vi "Parse Property Value.vi"(8 "error in":errorcluster, 10 "Property Type":T1, 11 "Node in":refnum<k20>) -> (0 "error out":errorcluster, 2 "Property Value":variant, 3 "Node out":refnum<k20>)   [LabVIEW 2024, in "Parser.lvlib" / "Property.lvclass"]
uses:
  Property.lvclass
  Controls/Property Type.ctl
  Controls/DependentFile.ctl
  <vilib>/xml/Close Reference(Node).vi
  <resource>/objmgr/DOMUserDefRef.rc
  <vilib>/xml/NI_XML.lvlib
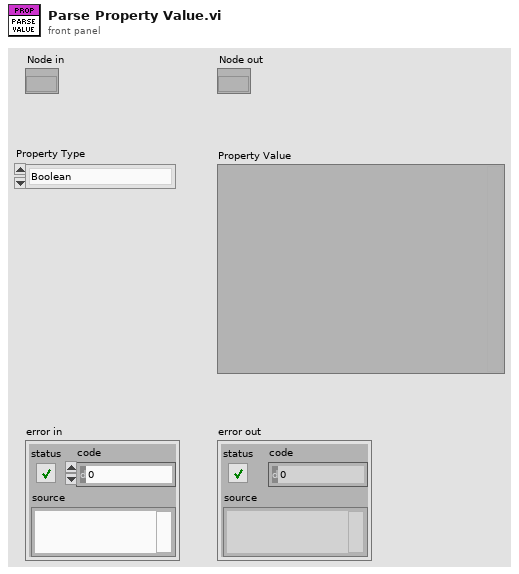
[diagram p1: front panel]
types:
  T1 = typedef "Parser.lvlib/Property.lvclass/Property Type.ctl" = enum16{"Boolean", "Double", "String", "Path", "Dictionary", "DependentFile", "I16", "I32", "I64", "U16", "U32", "U64", "BooleanArray", "DoubleArray", "StringArray", "I16Array", "I32Array", "I64Array", "U16Array", "U32Array", "U64Array", "Variant"}
  T2 = typedef "Parser.lvlib/Property.lvclass/DependentFile.ctl" = cluster{"Path":path, "Version":string, "RTDestination":path, "ForceDownload":bool, "SupportedTarget":string, "MD5":string, " Type":string}
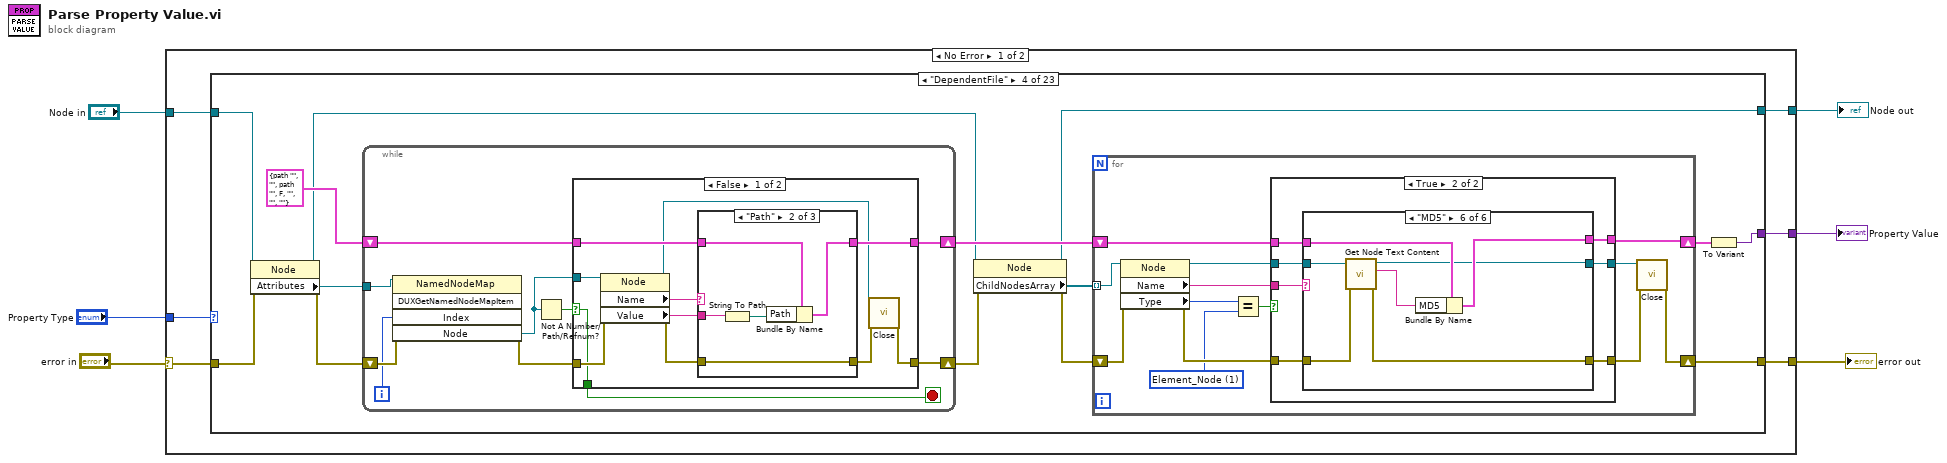
[diagram p0: block diagram]
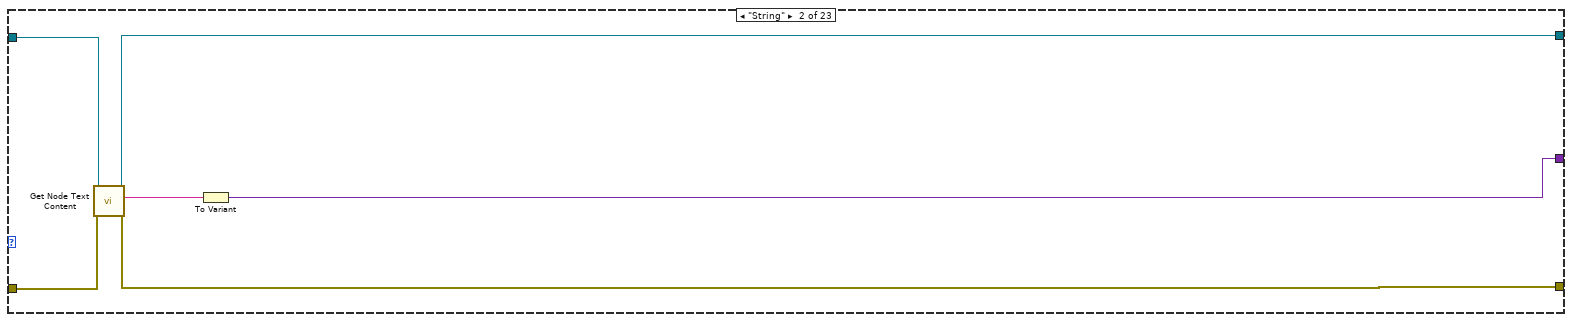
[diagram p3: hidden frame]
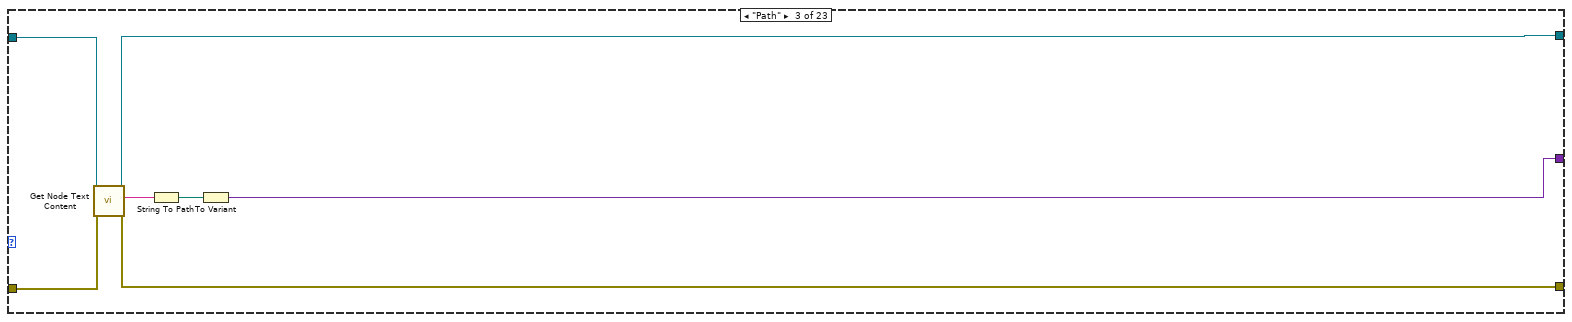
[diagram p4: hidden frame]
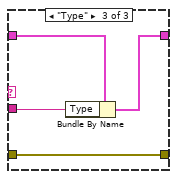
[diagram p6: hidden frame]
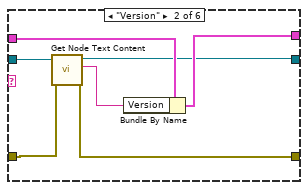
[diagram p10: hidden frame]
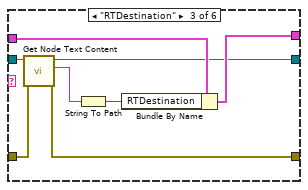
[diagram p11: hidden frame]
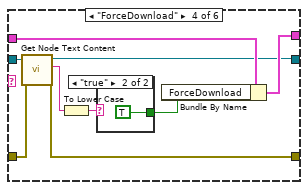
[diagram p12: hidden frame]
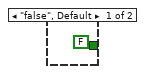
[diagram p13: hidden frame]
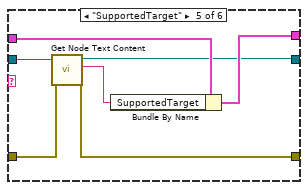
[diagram p14: hidden frame]
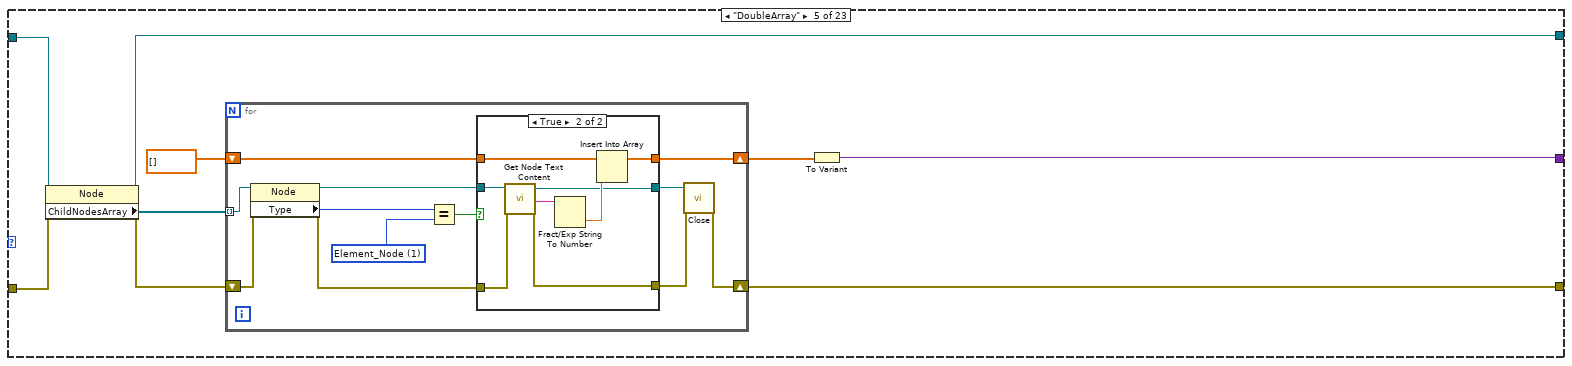
[diagram p15: hidden frame]
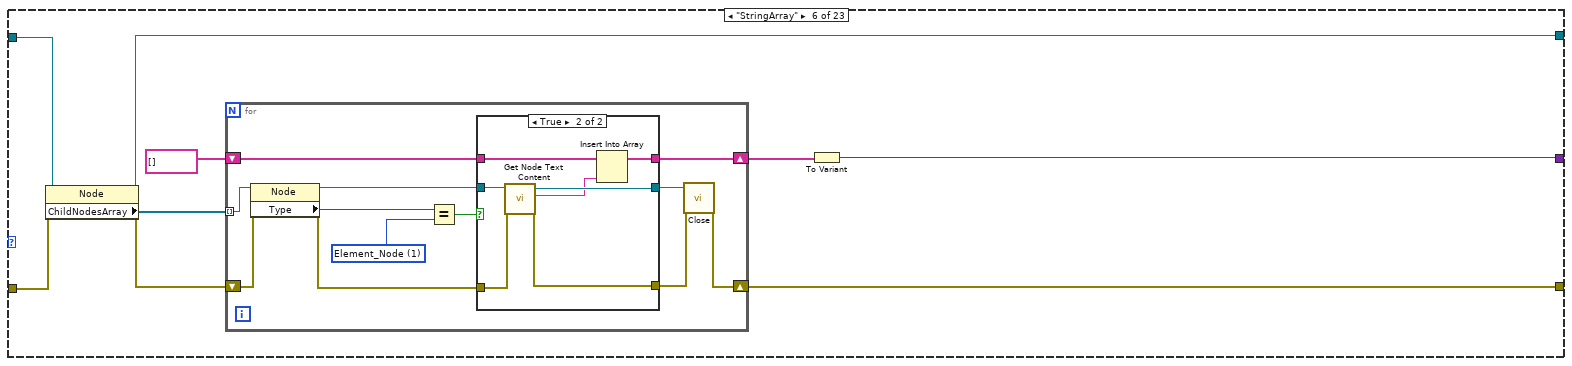
[diagram p17: hidden frame]
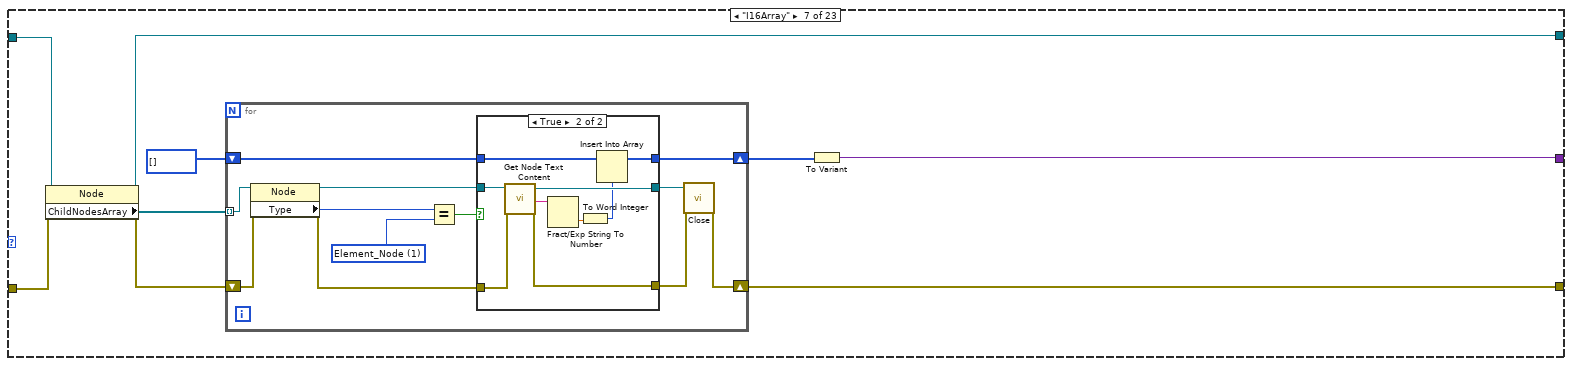
[diagram p19: hidden frame]
diagram:
  n1 = case shown="No Error" "error in" {
    selector: "error in" -> [w11 w608]
    tunnel: [w12 w608] -> w6
    tunnel: "Node in" -> [w10 w607]
    tunnel: [w9 _] -> w3
    tunnel: [w8 w607] -> w2
    tunnel: "Property Type" -> [w7 _]
    frame No Error {
      n2 = case shown="\"DependentFile\"" w7 {
        tunnel: w10 -> [w13 w16 w24 w36 w144 w176 w207 w240 w273 w306 w339 w372 w405 w439 w484 w492 w500 w508 w516 w524 w532 w539 w544]
        tunnel: [_ w18 w25 w35 w146 w178 w209 w242 w275 w308 w341 w374 w407 w441 w479 w487 w495 w503 w511 w519 w529 w536 w546] -> w9
        tunnel: w11 -> [w14 w20 w27 w41 w148 w180 w211 w244 w277 w310 w343 w376 w409 w443 w486 w494 w502 w510 w518 w526 w534 w541 w550]
        tunnel: [w14 w19 w26 w37 w150 w182 w213 w246 w279 w312 w345 w378 w411 w444 w485 w493 w501 w509 w517 w525 w533 w540 w548] -> w12
        tunnel: [w13 w15 w23 w29 w142 w174 w205 w238 w271 w304 w337 w370 w403 w436 w483 w491 w499 w507 w515 w523 w531 w538 w542] -> w8
        frame Default {
        }
        frame "String" {
          n3 = call <vilib>:"Get Node Text Content.vi"("error in (no error)"=w20, "node in"=w16) -> ("error out"=w19:errorcluster, "node text"=w17:string, "node out"=w15:refnum<k20>)  [unwired: 7 in]
          n4 = To Variant(anything=w17) -> (Variant=w18:variant)
        }
        frame "Path" {
          n5 = call <vilib>:"Get Node Text Content.vi"("error in (no error)"=w27, "node in"=w24) -> ("error out"=w26:errorcluster, "node text"=w22:string, "node out"=w23:refnum<k20>)  [unwired: 7 in]
          n6 = String To Path(string=w22) -> (path=w21:path)
          n7 = To Variant(anything=w21) -> (Variant=w25:variant)
        }
        frame "DependentFile" {
          n8 = property on="Property Node" class="Node"(reference=w36, error in=w41) -> (reference out=w30:refnum<k20>, error out=w40:errorcluster, "Attributes"=w34:refnum<k20>)
          n9 = while {
            tunnel: w34 -> [w48]
            shift-right: [w49] -> w39
            shift-left: w40 -> [w51]
            shift-right: [w44] -> w33
            shift-left: T2 {"Path"=path "", "Version"="", "RTDestination"=path "", "ForceDownload"=FALSE, "SupportedTarget"="", "MD5"="", " Type"=""} ("DependentFile") -> [w45]
            i -> [w47]
            stop <- w42 stop-if-true
            n10 = invoke on="Invoke Node" class="NamedNodeMap" method="DUXGetNamedNodeMapItem"(reference=w48, error in=w51, "Index"=w47) -> (error out=w50:errorcluster, "Node"=w43:refnum<k20>)  [unwired: 2 in, 3 out]
            n11 = Not A Number/Path/Refnum?(number/path/refnum=w43) -> (NaN/Path/Refnum?=w46:bool)
            n12 = case shown="False" w46 {
              selector: w46 -> [w52 w75]
              tunnel: w50 -> [w62 w76]
              tunnel: [w59 w76] -> w49
              tunnel: w43 -> [w58 _]
              tunnel: [w52 w75] -> w42
              tunnel: w45 -> [w56 w74]
              tunnel: [w55 w74] -> w44
              frame False {
                n13 = property on="Property Node" class="Node"(reference=w58, error in=w62) -> (reference out=w54:refnum<k20>, error out=w61:errorcluster, "Name"=w57:string, "Value"=w53:string)
                n14 = case shown="\"Path\"" w57 {
                  tunnel: w56 -> [w63 w68 w72]
                  tunnel: [w63 w67 w71] -> w55
                  tunnel: w61 -> [w64 w69 w73]
                  tunnel: [w64 w69 w73] -> w60
                  tunnel: w53 -> [_ w65 w70]
                  frame "-1", Default {
                  }
                  frame "Path" {
                    n15 = String To Path(string=w65) -> (path=w66:path)
                    n16 = Bundle By Name(cluster=w68, "Path"=w66) -> (w67:T2)
                  }
                  frame "Type" {
                    n17 = Bundle By Name(cluster=w72, "Type"=w70) -> (w71:T2)
                  }
                }
                n18 = call-poly <vilib>:"Close.vi"("error in (no error)"=w60, "node"=w54) -> ("error out"=w59:errorcluster)  [unwired: 7 in]
              }
              frame True {
              }
            }
          }
          n19 = property class="Node"(reference=w30, error in=w39) -> (reference out=w29:refnum<k20>, error out=w38:errorcluster, "ChildNodesArray"=w28:refnum<k20>[])
          n20 = for {
            shift-right: [w87] -> w37
            shift-left: w38 -> [w89]
            shift-right: [w82] -> w32
            shift-left: w33 -> [w84]
            tunnel: w28 -> [w80] mode=indexing
            w77 = 1 items=["Element_Node"=1, "Attribute_Node"=2, "Text_Node"=3, "CDATASection_Node"=4, "EntityReference_Node"=5, "Entity_Node"=6, "ProcessingInstruction_Node"=7, "Comment_Node"=8, "Document_Node"=9, "DocumentType_Node"=10, "DocumentFragment_Node"=11, "Notation_Node"=12] ("Node Type")
            n21 = property on="Property Node" class="Node"(reference=w80, error in=w89) -> (reference out=w83:refnum<k20>, error out=w86:errorcluster, "Name"=w85:string, "Type"=w79:i32)
            n22 = Equal?(x=w79, y=w77) -> (x = y?=w78:bool)
            n23 = case shown="True" w78 {
              tunnel: w85 -> [_ w97]
              tunnel: w84 -> [w90 w96]
              tunnel: w83 -> [w91 w95]
              tunnel: [w90 w94] -> w82
              tunnel: [w92 w99] -> w88
              tunnel: [w91 w93] -> w81
              tunnel: w86 -> [w92 w98]
              frame False {
              }
              frame True {
                n24 = case shown="\"MD5\"" w97 {
                  tunnel: w96 -> [w101 w106 w114 w123 w132 w139]
                  tunnel: w95 -> [w100 w105 w113 w122 w131 w138]
                  tunnel: [w101 w104 w111 w118 w129 w136] -> w94
                  tunnel: [_ w108 w116 w125 w134 w141] -> w99
                  tunnel: [w100 w103 w110 w117 w128 w135] -> w93
                  tunnel: w98 -> [_ w107 w115 w124 w133 w140]
                  frame "-1", Default {
                  }
                  frame "Version" {
                    n25 = call <vilib>:"Get Node Text Content.vi"("error in (no error)"=w107, "node in"=w105) -> ("error out"=w108:errorcluster, "node text"=w102:string, "node out"=w103:refnum<k20>)  [unwired: 7 in]
                    n26 = Bundle By Name(cluster=w106, "Version"=w102) -> (w104:T2)
                  }
                  frame "RTDestination" {
                    n27 = call <vilib>:"Get Node Text Content.vi"("error in (no error)"=w115, "node in"=w113) -> ("error out"=w116:errorcluster, "node text"=w112:string, "node out"=w110:refnum<k20>)  [unwired: 7 in]
                    n28 = String To Path(string=w112) -> (path=w109:path)
                    n29 = Bundle By Name(cluster=w114, "RTDestination"=w109) -> (w111:T2)
                  }
                  frame "ForceDownload" {
                    n30 = call <vilib>:"Get Node Text Content.vi"("error in (no error)"=w124, "node in"=w122) -> ("error out"=w125:errorcluster, "node text"=w121:string, "node out"=w117:refnum<k20>)  [unwired: 7 in]
                    n31 = To Lower Case(string=w121) -> (all lower case string=w120:string)
                    n32 = case shown="\"true\"" w120 {
                      tunnel: [FALSE ("ForceDownload") TRUE ("ForceDownload")] -> w119
                      frame "false", Default {
                      }
                      frame "true" {
                      }
                    }
                    n33 = Bundle By Name(cluster=w123, "ForceDownload"=w119) -> (w118:T2)
                  }
                  frame "SupportedTarget" {
                    n34 = call <vilib>:"Get Node Text Content.vi"("error in (no error)"=w133, "node in"=w131) -> ("error out"=w134:errorcluster, "node text"=w130:string, "node out"=w128:refnum<k20>)  [unwired: 7 in]
                    n35 = Bundle By Name(cluster=w132, "SupportedTarget"=w130) -> (w129:T2)
                  }
                  frame "MD5" {
                    n36 = call <vilib>:"Get Node Text Content.vi"("error in (no error)"=w140, "node in"=w138) -> ("error out"=w141:errorcluster, "node text"=w137:string, "node out"=w135:refnum<k20>)  [unwired: 7 in]
                    n37 = Bundle By Name(cluster=w139, "MD5"=w137) -> (w136:T2)
                  }
                }
              }
            }
            n38 = call-poly <vilib>:"Close.vi"("error in (no error)"=w88, "node"=w81) -> ("error out"=w87:errorcluster)  [unwired: 7 in]
          }
          n39 = To Variant(anything=w32) -> (Variant=w35:variant)
        }
        frame "DoubleArray" {
          n40 = property class="Node"(reference=w144, error in=w148) -> (reference out=w142:refnum<k20>, error out=w149:errorcluster, "ChildNodesArray"=w143:refnum<k20>[])
          n41 = for {
            shift-right: [w153] -> w145
            shift-left: dbl[] [] -> [w155]
            shift-right: [w159] -> w150
            shift-left: w149 -> [w162]
            tunnel: w143 -> [w157] mode=indexing
            w158 = 1 items=["Element_Node"=1, "Attribute_Node"=2, "Text_Node"=3, "CDATASection_Node"=4, "EntityReference_Node"=5, "Entity_Node"=6, "ProcessingInstruction_Node"=7, "Comment_Node"=8, "Document_Node"=9, "DocumentType_Node"=10, "DocumentFragment_Node"=11, "Notation_Node"=12] ("Node Type")
            n42 = property class="Node"(reference=w157, error in=w162) -> (reference out=w152:refnum<k20>, error out=w161:errorcluster, "Type"=w156:i32)
            n43 = Equal?(x=w156, y=w158) -> (x = y?=w154:bool)
            n44 = case shown="True" w154 {
              tunnel: [w165 w172] -> w160
              tunnel: w155 -> [w164 w166]
              tunnel: [w164 w170] -> w153
              tunnel: w161 -> [w165 w173]
              tunnel: w152 -> [w163 w169]
              tunnel: [w163 w167] -> w151
              frame False {
              }
              frame True {
                n45 = call <vilib>:"Get Node Text Content.vi"("error in (no error)"=w173, "node in"=w169) -> ("error out"=w172:errorcluster, "node text"=w171:string, "node out"=w167:refnum<k20>)  [unwired: 7 in]
                n46 = Fract/Exp String To Number(string=w171) -> (number=w168:dbl)  [unwired: 3 in, 1 out]
                n47 = Insert Into Array(array=w166, new element=w168) -> (w170:dbl[])  [unwired: 1 in]
              }
            }
            n48 = call-poly <vilib>:"Close.vi"("error in (no error)"=w160, "node"=w151) -> ("error out"=w159:errorcluster)  [unwired: 7 in]
          }
          n49 = To Variant(anything=w145) -> (Variant=w146:variant)
        }
        frame "StringArray" {
          n50 = property class="Node"(reference=w176, error in=w180) -> (reference out=w174:refnum<k20>, error out=w181:errorcluster, "ChildNodesArray"=w175:refnum<k20>[])
          n51 = for {
            shift-right: [w185] -> w177
            shift-left: string[] [] -> [w187]
            shift-right: [w191] -> w182
            shift-left: w181 -> [w194]
            tunnel: w175 -> [w189] mode=indexing
            w190 = 1 items=["Element_Node"=1, "Attribute_Node"=2, "Text_Node"=3, "CDATASection_Node"=4, "EntityReference_Node"=5, "Entity_Node"=6, "ProcessingInstruction_Node"=7, "Comment_Node"=8, "Document_Node"=9, "DocumentType_Node"=10, "DocumentFragment_Node"=11, "Notation_Node"=12] ("Node Type")
            n52 = property class="Node"(reference=w189, error in=w194) -> (reference out=w184:refnum<k20>, error out=w193:errorcluster, "Type"=w188:i32)
            n53 = Equal?(x=w188, y=w190) -> (x = y?=w186:bool)
            n54 = case shown="True" w186 {
              tunnel: [w197 w203] -> w192
              tunnel: w187 -> [w196 w199]
              tunnel: [w196 w202] -> w185
              tunnel: w193 -> [w197 w204]
              tunnel: w184 -> [w195 w201]
              tunnel: [w195 w200] -> w183
              frame False {
              }
              frame True {
                n55 = call <vilib>:"Get Node Text Content.vi"("error in (no error)"=w204, "node in"=w201) -> ("error out"=w203:errorcluster, "node text"=w198:string, "node out"=w200:refnum<k20>)  [unwired: 7 in]
                n56 = Insert Into Array(array=w199, new element=w198) -> (w202:string[])  [unwired: 1 in]
              }
            }
            n57 = call-poly <vilib>:"Close.vi"("error in (no error)"=w192, "node"=w183) -> ("error out"=w191:errorcluster)  [unwired: 7 in]
          }
          n58 = To Variant(anything=w177) -> (Variant=w178:variant)
        }
        frame "I16Array" {
          n59 = property class="Node"(reference=w207, error in=w211) -> (reference out=w205:refnum<k20>, error out=w212:errorcluster, "ChildNodesArray"=w206:refnum<k20>[])
          n60 = for {
            shift-right: [w216] -> w208
            shift-left: i16[] [] -> [w218]
            shift-right: [w222] -> w213
            shift-left: w212 -> [w225]
            tunnel: w206 -> [w220] mode=indexing
            w221 = 1 items=["Element_Node"=1, "Attribute_Node"=2, "Text_Node"=3, "CDATASection_Node"=4, "EntityReference_Node"=5, "Entity_Node"=6, "ProcessingInstruction_Node"=7, "Comment_Node"=8, "Document_Node"=9, "DocumentType_Node"=10, "DocumentFragment_Node"=11, "Notation_Node"=12] ("Node Type")
            n61 = property class="Node"(reference=w220, error in=w225) -> (reference out=w215:refnum<k20>, error out=w224:errorcluster, "Type"=w219:i32)
            n62 = Equal?(x=w219, y=w221) -> (x = y?=w217:bool)
            n63 = case shown="True" w217 {
              tunnel: [w228 w236] -> w223
              tunnel: w218 -> [w227 w231]
              tunnel: [w227 w234] -> w216
              tunnel: w224 -> [w228 w237]
              tunnel: w215 -> [w226 w233]
              tunnel: [w226 w232] -> w214
              frame False {
              }
              frame True {
                n64 = call <vilib>:"Get Node Text Content.vi"("error in (no error)"=w237, "node in"=w233) -> ("error out"=w236:errorcluster, "node text"=w235:string, "node out"=w232:refnum<k20>)  [unwired: 7 in]
                n65 = Fract/Exp String To Number(string=w235) -> (number=w230:dbl)  [unwired: 3 in, 1 out]
                n66 = To Word Integer(number=w230) -> (16bit integer=w229:i16)
                n67 = Insert Into Array(array=w231, new element=w229) -> (w234:i16[])  [unwired: 1 in]
              }
            }
            n68 = call-poly <vilib>:"Close.vi"("error in (no error)"=w223, "node"=w214) -> ("error out"=w222:errorcluster)  [unwired: 7 in]
          }
          n69 = To Variant(anything=w208) -> (Variant=w209:variant)
        }
        frame "I32Array" {
          n70 = property class="Node"(reference=w240, error in=w244) -> (reference out=w238:refnum<k20>, error out=w245:errorcluster, "ChildNodesArray"=w239:refnum<k20>[])
          n71 = for {
            shift-right: [w249] -> w241
            shift-left: i32[] [] -> [w251]
            shift-right: [w255] -> w246
            shift-left: w245 -> [w258]
            tunnel: w239 -> [w253] mode=indexing
            w254 = 1 items=["Element_Node"=1, "Attribute_Node"=2, "Text_Node"=3, "CDATASection_Node"=4, "EntityReference_Node"=5, "Entity_Node"=6, "ProcessingInstruction_Node"=7, "Comment_Node"=8, "Document_Node"=9, "DocumentType_Node"=10, "DocumentFragment_Node"=11, "Notation_Node"=12] ("Node Type")
            n72 = property class="Node"(reference=w253, error in=w258) -> (reference out=w248:refnum<k20>, error out=w257:errorcluster, "Type"=w252:i32)
            n73 = Equal?(x=w252, y=w254) -> (x = y?=w250:bool)
            n74 = case shown="True" w250 {
              tunnel: [w261 w269] -> w256
              tunnel: w251 -> [w260 w263]
              tunnel: [w260 w267] -> w249
              tunnel: w257 -> [w261 w270]
              tunnel: w248 -> [w259 w266]
              tunnel: [w259 w264] -> w247
              frame False {
              }
              frame True {
                n75 = call <vilib>:"Get Node Text Content.vi"("error in (no error)"=w270, "node in"=w266) -> ("error out"=w269:errorcluster, "node text"=w268:string, "node out"=w264:refnum<k20>)  [unwired: 7 in]
                n76 = Fract/Exp String To Number(string=w268) -> (number=w265:dbl)  [unwired: 3 in, 1 out]
                n77 = To Long Integer(number=w265) -> (32bit integer=w262:i32)
                n78 = Insert Into Array(array=w263, new element=w262) -> (w267:i32[])  [unwired: 1 in]
              }
            }
            n79 = call-poly <vilib>:"Close.vi"("error in (no error)"=w256, "node"=w247) -> ("error out"=w255:errorcluster)  [unwired: 7 in]
          }
          n80 = To Variant(anything=w241) -> (Variant=w242:variant)
        }
        frame "I64Array" {
          n81 = property class="Node"(reference=w273, error in=w277) -> (reference out=w271:refnum<k20>, error out=w278:errorcluster, "ChildNodesArray"=w272:refnum<k20>[])
          n82 = for {
            shift-right: [w282] -> w274
            shift-left: i64[] [] -> [w284]
            shift-right: [w288] -> w279
            shift-left: w278 -> [w291]
            tunnel: w272 -> [w286] mode=indexing
            w287 = 1 items=["Element_Node"=1, "Attribute_Node"=2, "Text_Node"=3, "CDATASection_Node"=4, "EntityReference_Node"=5, "Entity_Node"=6, "ProcessingInstruction_Node"=7, "Comment_Node"=8, "Document_Node"=9, "DocumentType_Node"=10, "DocumentFragment_Node"=11, "Notation_Node"=12] ("Node Type")
            n83 = property class="Node"(reference=w286, error in=w291) -> (reference out=w281:refnum<k20>, error out=w290:errorcluster, "Type"=w285:i32)
            n84 = Equal?(x=w285, y=w287) -> (x = y?=w283:bool)
            n85 = case shown="True" w283 {
              tunnel: [w294 w302] -> w289
              tunnel: w284 -> [w293 w296]
              tunnel: [w293 w300] -> w282
              tunnel: w290 -> [w294 w303]
              tunnel: w281 -> [w292 w299]
              tunnel: [w292 w297] -> w280
              frame False {
              }
              frame True {
                n86 = call <vilib>:"Get Node Text Content.vi"("error in (no error)"=w303, "node in"=w299) -> ("error out"=w302:errorcluster, "node text"=w301:string, "node out"=w297:refnum<k20>)  [unwired: 7 in]
                n87 = Fract/Exp String To Number(string=w301) -> (number=w298:dbl)  [unwired: 3 in, 1 out]
                n88 = To Quad Integer(1:w298) -> (0:w295:i64)
                n89 = Insert Into Array(array=w296, new element=w295) -> (w300:i64[])  [unwired: 1 in]
              }
            }
            n90 = call-poly <vilib>:"Close.vi"("error in (no error)"=w289, "node"=w280) -> ("error out"=w288:errorcluster)  [unwired: 7 in]
          }
          n91 = To Variant(anything=w274) -> (Variant=w275:variant)
        }
        frame "U16Array" {
          n92 = property class="Node"(reference=w306, error in=w310) -> (reference out=w304:refnum<k20>, error out=w311:errorcluster, "ChildNodesArray"=w305:refnum<k20>[])
          n93 = for {
            shift-right: [w315] -> w307
            shift-left: u16[] [] -> [w317]
            shift-right: [w321] -> w312
            shift-left: w311 -> [w324]
            tunnel: w305 -> [w319] mode=indexing
            w320 = 1 items=["Element_Node"=1, "Attribute_Node"=2, "Text_Node"=3, "CDATASection_Node"=4, "EntityReference_Node"=5, "Entity_Node"=6, "ProcessingInstruction_Node"=7, "Comment_Node"=8, "Document_Node"=9, "DocumentType_Node"=10, "DocumentFragment_Node"=11, "Notation_Node"=12] ("Node Type")
            n94 = property class="Node"(reference=w319, error in=w324) -> (reference out=w314:refnum<k20>, error out=w323:errorcluster, "Type"=w318:i32)
            n95 = Equal?(x=w318, y=w320) -> (x = y?=w316:bool)
            n96 = case shown="True" w316 {
              tunnel: [w327 w335] -> w322
              tunnel: w317 -> [w326 w329]
              tunnel: [w326 w333] -> w315
              tunnel: w323 -> [w327 w336]
              tunnel: w314 -> [w325 w332]
              tunnel: [w325 w330] -> w313
              frame False {
              }
              frame True {
                n97 = call <vilib>:"Get Node Text Content.vi"("error in (no error)"=w336, "node in"=w332) -> ("error out"=w335:errorcluster, "node text"=w334:string, "node out"=w330:refnum<k20>)  [unwired: 7 in]
                n98 = Fract/Exp String To Number(string=w334) -> (number=w331:dbl)  [unwired: 3 in, 1 out]
                n99 = To Unsigned Word Integer(number=w331) -> (unsigned 16bit integer=w328:u16)
                n100 = Insert Into Array(array=w329, new element=w328) -> (w333:u16[])  [unwired: 1 in]
              }
            }
            n101 = call-poly <vilib>:"Close.vi"("error in (no error)"=w322, "node"=w313) -> ("error out"=w321:errorcluster)  [unwired: 7 in]
          }
          n102 = To Variant(anything=w307) -> (Variant=w308:variant)
        }
        frame "U32Array" {
          n103 = property class="Node"(reference=w339, error in=w343) -> (reference out=w337:refnum<k20>, error out=w344:errorcluster, "ChildNodesArray"=w338:refnum<k20>[])
          n104 = for {
            shift-right: [w348] -> w340
            shift-left: u32[] [] -> [w350]
            shift-right: [w354] -> w345
            shift-left: w344 -> [w357]
            tunnel: w338 -> [w352] mode=indexing
            w353 = 1 items=["Element_Node"=1, "Attribute_Node"=2, "Text_Node"=3, "CDATASection_Node"=4, "EntityReference_Node"=5, "Entity_Node"=6, "ProcessingInstruction_Node"=7, "Comment_Node"=8, "Document_Node"=9, "DocumentType_Node"=10, "DocumentFragment_Node"=11, "Notation_Node"=12] ("Node Type")
            n105 = property class="Node"(reference=w352, error in=w357) -> (reference out=w347:refnum<k20>, error out=w356:errorcluster, "Type"=w351:i32)
            n106 = Equal?(x=w351, y=w353) -> (x = y?=w349:bool)
            n107 = case shown="True" w349 {
              tunnel: [w360 w368] -> w355
              tunnel: w350 -> [w359 w362]
              tunnel: [w359 w366] -> w348
              tunnel: w356 -> [w360 w369]
              tunnel: w347 -> [w358 w365]
              tunnel: [w358 w363] -> w346
              frame False {
              }
              frame True {
                n108 = call <vilib>:"Get Node Text Content.vi"("error in (no error)"=w369, "node in"=w365) -> ("error out"=w368:errorcluster, "node text"=w367:string, "node out"=w363:refnum<k20>)  [unwired: 7 in]
                n109 = Fract/Exp String To Number(string=w367) -> (number=w364:dbl)  [unwired: 3 in, 1 out]
                n110 = To Unsigned Long Integer(number=w364) -> (unsigned 32bit integer=w361:u32)
                n111 = Insert Into Array(array=w362, new element=w361) -> (w366:u32[])  [unwired: 1 in]
              }
            }
            n112 = call-poly <vilib>:"Close.vi"("error in (no error)"=w355, "node"=w346) -> ("error out"=w354:errorcluster)  [unwired: 7 in]
          }
          n113 = To Variant(anything=w340) -> (Variant=w341:variant)
        }
        frame "U64Array" {
          n114 = property class="Node"(reference=w372, error in=w376) -> (reference out=w370:refnum<k20>, error out=w377:errorcluster, "ChildNodesArray"=w371:refnum<k20>[])
          n115 = for {
            shift-right: [w381] -> w373
            shift-left: u64[] [] -> [w383]
            shift-right: [w387] -> w378
            shift-left: w377 -> [w390]
            tunnel: w371 -> [w385] mode=indexing
            w386 = 1 items=["Element_Node"=1, "Attribute_Node"=2, "Text_Node"=3, "CDATASection_Node"=4, "EntityReference_Node"=5, "Entity_Node"=6, "ProcessingInstruction_Node"=7, "Comment_Node"=8, "Document_Node"=9, "DocumentType_Node"=10, "DocumentFragment_Node"=11, "Notation_Node"=12] ("Node Type")
            n116 = property class="Node"(reference=w385, error in=w390) -> (reference out=w380:refnum<k20>, error out=w389:errorcluster, "Type"=w384:i32)
            n117 = Equal?(x=w384, y=w386) -> (x = y?=w382:bool)
            n118 = case shown="True" w382 {
              tunnel: [w393 w401] -> w388
              tunnel: w383 -> [w392 w395]
              tunnel: [w392 w399] -> w381
              tunnel: w389 -> [w393 w402]
              tunnel: w380 -> [w391 w398]
              tunnel: [w391 w396] -> w379
              frame False {
              }
              frame True {
                n119 = call <vilib>:"Get Node Text Content.vi"("error in (no error)"=w402, "node in"=w398) -> ("error out"=w401:errorcluster, "node text"=w400:string, "node out"=w396:refnum<k20>)  [unwired: 7 in]
                n120 = Fract/Exp String To Number(string=w400) -> (number=w397:dbl)  [unwired: 3 in, 1 out]
                n121 = To Unsigned Quad Integer(1:w397) -> (0:w394:u64)
                n122 = Insert Into Array(array=w395, new element=w394) -> (w399:u64[])  [unwired: 1 in]
              }
            }
            n123 = call-poly <vilib>:"Close.vi"("error in (no error)"=w388, "node"=w379) -> ("error out"=w387:errorcluster)  [unwired: 7 in]
          }
          n124 = To Variant(anything=w373) -> (Variant=w374:variant)
        }
        frame "BooleanArray" {
          n125 = property class="Node"(reference=w405, error in=w409) -> (reference out=w403:refnum<k20>, error out=w410:errorcluster, "ChildNodesArray"=w404:refnum<k20>[])
          n126 = for {
            shift-right: [w414] -> w406
            shift-left: bool[] [] -> [w416]
            shift-right: [w420] -> w411
            shift-left: w410 -> [w423]
            tunnel: w404 -> [w418] mode=indexing
            w419 = 1 items=["Element_Node"=1, "Attribute_Node"=2, "Text_Node"=3, "CDATASection_Node"=4, "EntityReference_Node"=5, "Entity_Node"=6, "ProcessingInstruction_Node"=7, "Comment_Node"=8, "Document_Node"=9, "DocumentType_Node"=10, "DocumentFragment_Node"=11, "Notation_Node"=12] ("Node Type")
            n127 = property class="Node"(reference=w418, error in=w423) -> (reference out=w413:refnum<k20>, error out=w422:errorcluster, "Type"=w417:i32)
            n128 = Equal?(x=w417, y=w419) -> (x = y?=w415:bool)
            n129 = case shown="True" w415 {
              tunnel: [w426 w434] -> w421
              tunnel: w416 -> [w425 w429]
              tunnel: [w425 w432] -> w414
              tunnel: w422 -> [w426 w435]
              tunnel: w413 -> [w424 w431]
              tunnel: [w424 w430] -> w412
              frame False {
              }
              frame True {
                n130 = call <vilib>:"Get Node Text Content.vi"("error in (no error)"=w435, "node in"=w431) -> ("error out"=w434:errorcluster, "node text"=w433:string, "node out"=w430:refnum<k20>)  [unwired: 7 in]
                n131 = Fract/Exp String To Number(string=w433) -> (number=w428:dbl)  [unwired: 3 in, 1 out]
                n132 = Not Equal To 0?(x=w428) -> (x != 0?=w427:bool)
                n133 = Insert Into Array(array=w429, new element=w427) -> (w432:bool[])  [unwired: 1 in]
              }
            }
            n134 = call-poly <vilib>:"Close.vi"("error in (no error)"=w421, "node"=w412) -> ("error out"=w420:errorcluster)  [unwired: 7 in]
          }
          n135 = To Variant(anything=w406) -> (Variant=w407:variant)
        }
        frame "Variant" {
          n136 = property class="Node"(reference=w439, error in=w443) -> (reference out=w436:refnum<k20>, error out=w442:errorcluster, "ChildNodesArray"=w437:refnum<k20>[])
          n137 = for {
            tunnel: w437 -> [w450] mode=indexing
            shift-right: [w451] -> w440
            shift-left: cluster{"Type":u8[], "Data":u8[]} {"Type"=[], "Data"=[]} -> [w452]
            shift-right: [w455] -> w444
            shift-left: w442 -> [w454]
            w449 = 1 items=["Element_Node"=1, "Attribute_Node"=2, "Text_Node"=3, "CDATASection_Node"=4, "EntityReference_Node"=5, "Entity_Node"=6, "ProcessingInstruction_Node"=7, "Comment_Node"=8, "Document_Node"=9, "DocumentType_Node"=10, "DocumentFragment_Node"=11, "Notation_Node"=12] ("Node Type")
            n138 = property class="Node"(reference=w450, error in=w454) -> (reference out=w445:refnum<k20>, error out=w453:errorcluster, "Name"=w446:string, "Type"=w448:i32)
            n139 = Equal?(x=w448, y=w449) -> (x = y?=w447:bool)
            n140 = case shown="True" w447 {
              tunnel: w453 -> [w457 w468]
              tunnel: [w457 w467] -> w455
              tunnel: w452 -> [w456 w464]
              tunnel: [w456 w461] -> w451
              tunnel: w446 -> [_ w460]
              tunnel: w445 -> [_ w459]
              frame False {
              }
              frame True {
                n141 = call <vilib>:"Get Node Text Content.vi"("error in (no error)"=w468, "node in"=w459) -> ("error out"=w465:errorcluster, "node text"=w463:string, "node out"=w458:refnum<k20>)  [unwired: 7 in]
                n142 = String To Byte Array(string=w463) -> (unsigned byte array=w462:u8[])
                n143 = case shown="\"Data\"" w460 {
                  tunnel: w464 -> [w469 w473 w477]
                  tunnel: w462 -> [_ w472 w476]
                  tunnel: [w469 w471 w475] -> w461
                  tunnel: w465 -> [w470 w474 w478]
                  tunnel: [w470 w474 w478] -> w466
                  frame "-1", Default {
                  }
                  frame "Type" {
                    n144 = Bundle By Name(cluster=w473, "Type"=w472) -> (w471:cluster{"Type":u8[], "Data":u8[]})
                  }
                  frame "Data" {
                    n145 = Bundle By Name(cluster=w477, "Data"=w476) -> (w475:cluster{"Type":u8[], "Data":u8[]})
                  }
                }
                n146 = call-poly <vilib>:"Close.vi"("error in (no error)"=w466, "node"=w458) -> ("error out"=w467:errorcluster)  [unwired: 7 in]
              }
            }
          }
          n147 = To Variant(anything=w440) -> (Variant=w441:variant)
        }
        frame "U32" {
          n148 = call <vilib>:"Get Node Text Content.vi"("error in (no error)"=w486, "node in"=w484) -> ("error out"=w485:errorcluster, "node text"=w482:string, "node out"=w483:refnum<k20>)  [unwired: 7 in]
          n149 = Fract/Exp String To Number(string=w482) -> (number=w481:dbl)  [unwired: 3 in, 1 out]
          n150 = To Unsigned Long Integer(number=w481) -> (unsigned 32bit integer=w480:u32)
          n151 = To Variant(anything=w480) -> (Variant=w479:variant)
        }
        frame "U16" {
          n152 = call <vilib>:"Get Node Text Content.vi"("error in (no error)"=w494, "node in"=w492) -> ("error out"=w493:errorcluster, "node text"=w490:string, "node out"=w491:refnum<k20>)  [unwired: 7 in]
          n153 = Fract/Exp String To Number(string=w490) -> (number=w489:dbl)  [unwired: 3 in, 1 out]
          n154 = To Unsigned Word Integer(number=w489) -> (unsigned 16bit integer=w488:u16)
          n155 = To Variant(anything=w488) -> (Variant=w487:variant)
        }
        frame "U64" {
          n156 = call <vilib>:"Get Node Text Content.vi"("error in (no error)"=w502, "node in"=w500) -> ("error out"=w501:errorcluster, "node text"=w498:string, "node out"=w499:refnum<k20>)  [unwired: 7 in]
          n157 = Fract/Exp String To Number(string=w498) -> (number=w497:dbl)  [unwired: 3 in, 1 out]
          n158 = To Unsigned Quad Integer(1:w497) -> (0:w496:u64)
          n159 = To Variant(anything=w496) -> (Variant=w495:variant)
        }
        frame "I16" {
          n160 = call <vilib>:"Get Node Text Content.vi"("error in (no error)"=w510, "node in"=w508) -> ("error out"=w509:errorcluster, "node text"=w506:string, "node out"=w507:refnum<k20>)  [unwired: 7 in]
          n161 = Fract/Exp String To Number(string=w506) -> (number=w505:dbl)  [unwired: 3 in, 1 out]
          n162 = To Word Integer(number=w505) -> (16bit integer=w504:i16)
          n163 = To Variant(anything=w504) -> (Variant=w503:variant)
        }
        frame "I32" {
          n164 = call <vilib>:"Get Node Text Content.vi"("error in (no error)"=w518, "node in"=w516) -> ("error out"=w517:errorcluster, "node text"=w514:string, "node out"=w515:refnum<k20>)  [unwired: 7 in]
          n165 = Fract/Exp String To Number(string=w514) -> (number=w513:dbl)  [unwired: 3 in, 1 out]
          n166 = To Long Integer(number=w513) -> (32bit integer=w512:i32)
          n167 = To Variant(anything=w512) -> (Variant=w511:variant)
        }
        frame "I64" {
          n168 = call <vilib>:"Get Node Text Content.vi"("error in (no error)"=w526, "node in"=w524) -> ("error out"=w525:errorcluster, "node text"=w522:string, "node out"=w523:refnum<k20>)  [unwired: 7 in]
          n169 = Fract/Exp String To Number(string=w522) -> (number=w521:dbl)  [unwired: 3 in, 1 out]
          n170 = To Quad Integer(1:w521) -> (0:w520:i64)
          n171 = To Variant(anything=w520) -> (Variant=w519:variant)
        }
        frame "Boolean" {
          n172 = call <vilib>:"Get Node Text Content.vi"("error in (no error)"=w534, "node in"=w532) -> ("error out"=w533:errorcluster, "node text"=w530:string, "node out"=w531:refnum<k20>)  [unwired: 7 in]
          n173 = Fract/Exp String To Number(string=w530) -> (number=w527:dbl)  [unwired: 3 in, 1 out]
          n174 = Not Equal To 0?(x=w527) -> (x != 0?=w528:bool)
          n175 = To Variant(anything=w528) -> (Variant=w529:variant)
        }
        frame "Double" {
          n176 = call <vilib>:"Get Node Text Content.vi"("error in (no error)"=w541, "node in"=w539) -> ("error out"=w540:errorcluster, "node text"=w537:string, "node out"=w538:refnum<k20>)  [unwired: 7 in]
          n177 = Fract/Exp String To Number(string=w537) -> (number=w535:dbl)  [unwired: 3 in, 1 out]
          n178 = To Variant(anything=w535) -> (Variant=w536:variant)
        }
        frame "Dictionary" {
          w547 = map{string, dbl} {}  # Size: 0
          n179 = property class="Node"(reference=w544, error in=w550) -> (reference out=w542:refnum<k20>, error out=w549:errorcluster, "ChildNodesArray"=w543:refnum<k20>[])
          n180 = for {
            shift-right: [w557] -> w545
            shift-left: w547 -> [w558]
            tunnel: w543 -> [w556] mode=indexing
            shift-right: [w559] -> w548
            shift-left: w549 -> [w561]
            w555 = 1 items=["Element_Node"=1, "Attribute_Node"=2, "Text_Node"=3, "CDATASection_Node"=4, "EntityReference_Node"=5, "Entity_Node"=6, "ProcessingInstruction_Node"=7, "Comment_Node"=8, "Document_Node"=9, "DocumentType_Node"=10, "DocumentFragment_Node"=11, "Notation_Node"=12] ("Node Type")
            n181 = property class="Node"(reference=w556) -> (reference out=w551:refnum<k20>, "Type"=w554:i32)  [unwired: 1 in, 1 out]
            n182 = Equal?(x=w554, y=w555) -> (x = y?=w553:bool)
            n183 = case shown="True" w553 {
              tunnel: w561 -> [w564 w576]
              tunnel: w558 -> [w562 w572]
              tunnel: [w562 w571] -> w557
              tunnel: [w564 w574] -> w560
              tunnel: [w563 w566] -> w552
              tunnel: w551 -> [w563 w565]
              frame False {
              }
              frame True {
                n184 = property on="Property Node" class="Node"(reference=w565, error in=w576) -> (reference out=w567:refnum<k20>, error out=w577:errorcluster, "Attributes"=w573:refnum<k20>)
                n185 = invoke on="Invoke Node" class="NamedNodeMap" method="DUXGetNamedItem"(reference=w573, error in=w577, "Name"="Key") -> (error out=w575:errorcluster, "Node"=w569:refnum<k20>)  [unwired: 2 in, 3 out]
                n186 = Not A Number/Path/Refnum?(number/path/refnum=w569) -> (NaN/Path/Refnum?=w568:bool)
                n187 = case shown="False" w568 {
                  tunnel: w569 -> [w586 _]
                  tunnel: w567 -> [w585 w604]
                  tunnel: w572 -> [w583 w605]
                  tunnel: [w582 w605] -> w571
                  tunnel: w575 -> [w590 w606]
                  tunnel: [w587 w606] -> w574
                  tunnel: [w578 w604] -> w566
                  frame False {
                    n188 = call <vilib>:"Get Node Text Content.vi"("error in (no error)"=w590, "node in"=w586) -> ("error out"=w589:errorcluster, "node text"=w584:string, "node out"=w580:refnum<k20>)  [unwired: 7 in]
                    n189 = call <vilib>:"Get First Non-Text Child.vi"("error in (no error)"=w589, "node in"=w585) -> ("error out"=w591:errorcluster, "found child node?"=w579:bool, "child node"=w581:refnum<k20>, "node out"=w578:refnum<k20>)  [unwired: 6 in]
                    n190 = case shown="True" w579 {
                      tunnel: w591 -> [w593 w603]
                      tunnel: w584 -> [_ w600]
                      tunnel: w583 -> [w592 w599]
                      tunnel: [w592 w598] -> w582
                      tunnel: w581 -> [_ w597]
                      tunnel: [w593 w601] -> w588
                      frame False {
                      }
                      frame True {
                        n191 = call <vilib>:"Get Node Text Content.vi"("error in (no error)"=w603, "node in"=w597) -> ("error out"=w602:errorcluster, "node text"=w595:string, "node out"=w596:refnum<k20>)  [unwired: 7 in]
                        n192 = Fract/Exp String To Number(string=w595) -> (number=w594:dbl)  [unwired: 3 in, 1 out]
                        n193 = Insert Into Map(map in=w599, key=w600, value=w594) -> (map out=w598:map{string, dbl})  [unwired: 2 out]
                        n194 = call-poly <vilib>:"Close.vi"("error in (no error)"=w602, "node"=w596) -> ("error out"=w601:errorcluster)  [unwired: 7 in]
                      }
                    }
                    n195 = call-poly <vilib>:"Close.vi"("error in (no error)"=w588, "node"=w580) -> ("error out"=w587:errorcluster)  [unwired: 7 in]
                  }
                  frame True {
                  }
                }
              }
            }
            n196 = call-poly <vilib>:"Close.vi"("error in (no error)"=w560, "node"=w552) -> ("error out"=w559:errorcluster)  [unwired: 7 in]
          }
          n197 = To Variant(anything=w545) -> (Variant=w546:variant)
        }
      }
    }
    frame Error {
    }
  }
  "Property Value" <- w3
  "error out" <- w6
  "Node out" <- w2
